vi "OutBitsCheckSingleCMDSimpler.vi"(1 "scanChanged":bool, 2 "actScan":i32, 3 "stepChanged":bool, 4 "actStep":i32, 5 "outbit_in":bool, 9 "CMDin":u32) -> (19 "outbit_out":bool)   [LabVIEW 2014]
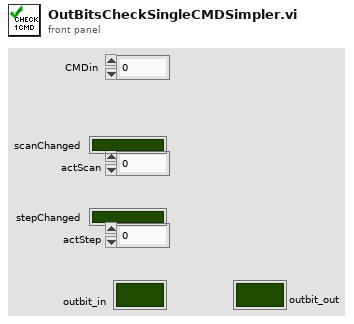
[diagram p1: front panel]
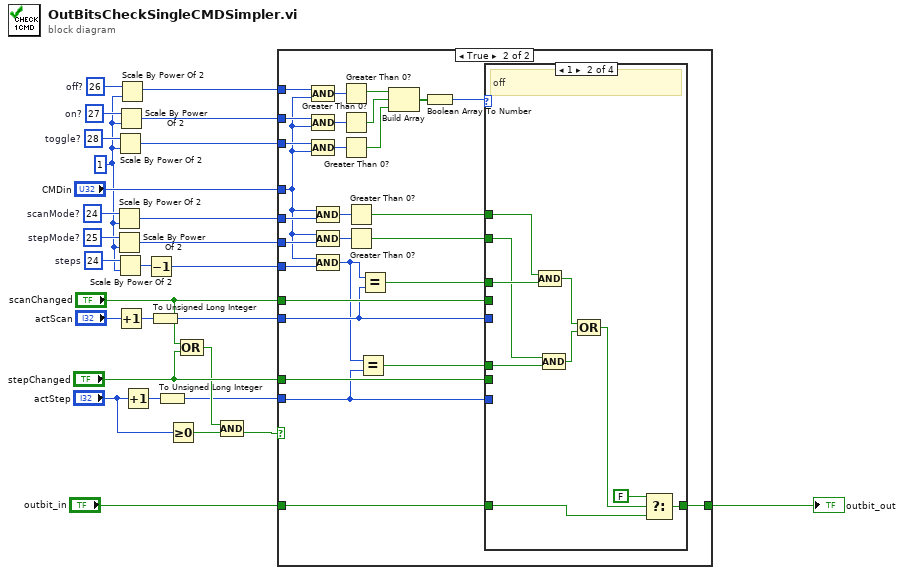
[diagram p0: block diagram]
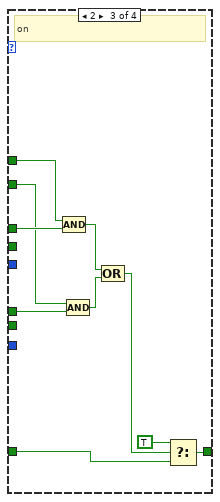
[diagram p4: hidden frame]
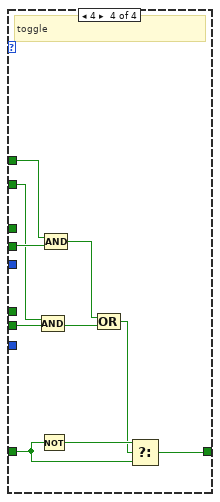
[diagram p5: hidden frame]
diagram:
  w15 = i16 24  # steps
  w16 = i16 25  # stepMode?
  w17 = i16 24  # scanMode?
  w26 = i16 26  # off?
  w27 = i16 27  # on?
  w14 = u32 1 ("Data")
  w28 = i16 28  # toggle?
  n1 = Scale By Power Of 2(n=w17, x=w14) -> (x*2^n=w10:u32)
  n2 = Scale By Power Of 2(n=w16, x=w14) -> (x*2^n=w11:u32)
  n3 = Scale By Power Of 2(n=w28, x=w14) -> (x*2^n=w19:u32)
  n4 = Scale By Power Of 2(n=w15, x=w14) -> (x*2^n=w13:u32)
  n5 = Scale By Power Of 2(n=w27, x=w14) -> (x*2^n=w21:u32)
  n6 = Increment(x="actScan") -> (x+1=w5:i32)
  n7 = Scale By Power Of 2(n=w26, x=w14) -> (x*2^n=w22:u32)
  n8 = Increment(x="actStep") -> (x+1=w2:i32)
  n9 = Decrement(x=w13) -> (x-1=w12:u32)
  n10 = To Unsigned Long Integer(number=w5) -> (unsigned 32bit integer=w4:u32)
  n11 = To Unsigned Long Integer(number=w2) -> (unsigned 32bit integer=w1:u32)
  n12 = Greater Or Equal To 0?(x="actStep") -> (x >= 0?=w25:bool)
  n13 = Compound Arithmetic op=OR("scanChanged", "stepChanged") -> (w6:bool)
  n14 = Compound Arithmetic op=AND(w6, w25) -> (w9:bool)
  n15 = case shown="True" w9 {
    tunnel: "CMDin" -> [_ w37]
    tunnel: w22 -> [_ w57]
    tunnel: w21 -> [_ w48]
    tunnel: "outbit_in" -> [w29 w45]
    tunnel: [w29 w46] -> w23
    tunnel: w19 -> [_ w47]
    tunnel: "scanChanged" -> [_ w44]
    tunnel: "stepChanged" -> [_ w43]
    tunnel: w1 -> [_ w34]
    tunnel: w4 -> [_ w36]
    tunnel: w12 -> [_ w38]
    tunnel: w11 -> [_ w39]
    tunnel: w10 -> [_ w40]
    frame False {
    }
    frame True {
      n16 = Compound Arithmetic op=AND(w57, w37) -> (w56:u32)
      n17 = Compound Arithmetic op=AND(w48, w37) -> (w55:u32)
      n18 = Compound Arithmetic op=AND(w47, w37) -> (w54:u32)
      n19 = Compound Arithmetic op=AND(w37, w40) -> (w42:u32)
      n20 = Compound Arithmetic op=AND(w37, w39) -> (w41:u32)
      n21 = Compound Arithmetic op=AND(w37, w38) -> (w35:u32)
      n22 = Greater Than 0?(x=w56) -> (x > 0?=w53:bool)
      n23 = Greater Than 0?(x=w55) -> (x > 0?=w52:bool)
      n24 = Greater Than 0?(x=w54) -> (x > 0?=w51:bool)
      n25 = Greater Than 0?(x=w42) -> (x > 0?=w31:bool)
      n26 = Greater Than 0?(x=w41) -> (x > 0?=w30:bool)
      n27 = Equal?(x=w35, y=w34) -> (x = y?=w33:bool)
      n28 = Equal?(x=w35, y=w36) -> (x = y?=w32:bool)
      n29 = Build Array(w53, w52, w51) -> (w50:bool[])
      n30 = Boolean Array To Number(Boolean array=w50) -> (number=w49:u8)
      n31 = case shown="1" w49 {
        tunnel: [w58 w62 w72 w86] -> w46
        tunnel: w45 -> [w58 w60 w70 w88]
        tunnel: w44 -> [_ _ _ w85]
        tunnel: w43 -> [_ _ _ w83]
        tunnel: w34 -> [_ _ _ _]
        tunnel: w36 -> [_ _ _ _]
        tunnel: w33 -> [_ w66 w76 _]
        tunnel: w32 -> [_ w67 w77 _]
        tunnel: w31 -> [_ w68 w78 w84]
        tunnel: w30 -> [_ w65 w75 w82]
        frame 0, Default {
        }
        frame 1 {
          # "off"
          n32 = Compound Arithmetic op=AND(w68, w67) -> (w64:bool)
          n33 = Compound Arithmetic op=AND(w65, w66) -> (w63:bool)
          n34 = Compound Arithmetic op=OR(w64, w63) -> (w61:bool)
          n35 = Select(t=FALSE, s=w61, f=w60) -> (s? t:f=w62:bool)
        }
        frame 2 {
          # "on"
          n36 = Compound Arithmetic op=AND(w78, w77) -> (w74:bool)
          n37 = Compound Arithmetic op=AND(w75, w76) -> (w73:bool)
          n38 = Compound Arithmetic op=OR(w74, w73) -> (w71:bool)
          n39 = Select(t=TRUE, s=w71, f=w70) -> (s? t:f=w72:bool)
        }
        frame 4 {
          # "toggle"
          n40 = Not(x=w88) -> (.not. x?=w87:bool)
          n41 = Compound Arithmetic op=AND(w82, w83) -> (w81:bool)
          n42 = Compound Arithmetic op=AND(w84, w85) -> (w80:bool)
          n43 = Compound Arithmetic op=OR(w80, w81) -> (w79:bool)
          n44 = Select(t=w87, s=w79, f=w88) -> (s? t:f=w86:bool)
        }
      }
    }
  }
  "outbit_out" <- w23
